vi "read groundwater header csv file.vi"(4 "Groundwater header file":path, 6 "header indicator reference 3":refnum<vi>, 7 "Groundwater Header":T1, 9 "Groundwater Cluster reference in":refnum<vi>, 10 "Read Groundwater Header File":bool, 11 "Sonde Serial Number String in":refnum<vi>) -> ()   [LabVIEW 2016]
uses:
  sdi_12/Groundwater header.ctl
  <vilib>/Utility/file.llb/Read Delimited Spreadsheet (string).vi
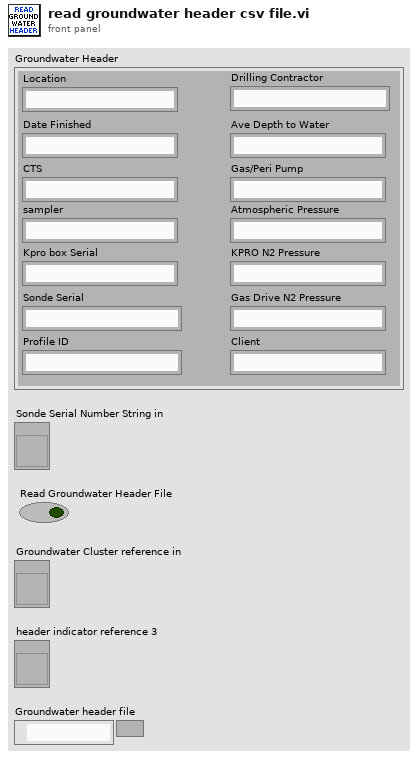
[diagram p1: front panel]
types:
  T1 = typedef "Groundwater header.ctl" = cluster{"Location":string, "Date Finished":string, "CTS":string, "sampler":string, "Kpro box Serial ":string, "Sonde Serial":string, "Drilling Contractor":string, "Ave Depth to Water":string, "Gas/Peri Pump":string, "Atmospheric Pressure":string, "KPRO N2 Pressure":string, "Gas Drive N2 Pressure":string, "Profile ID":string, "Client":string}
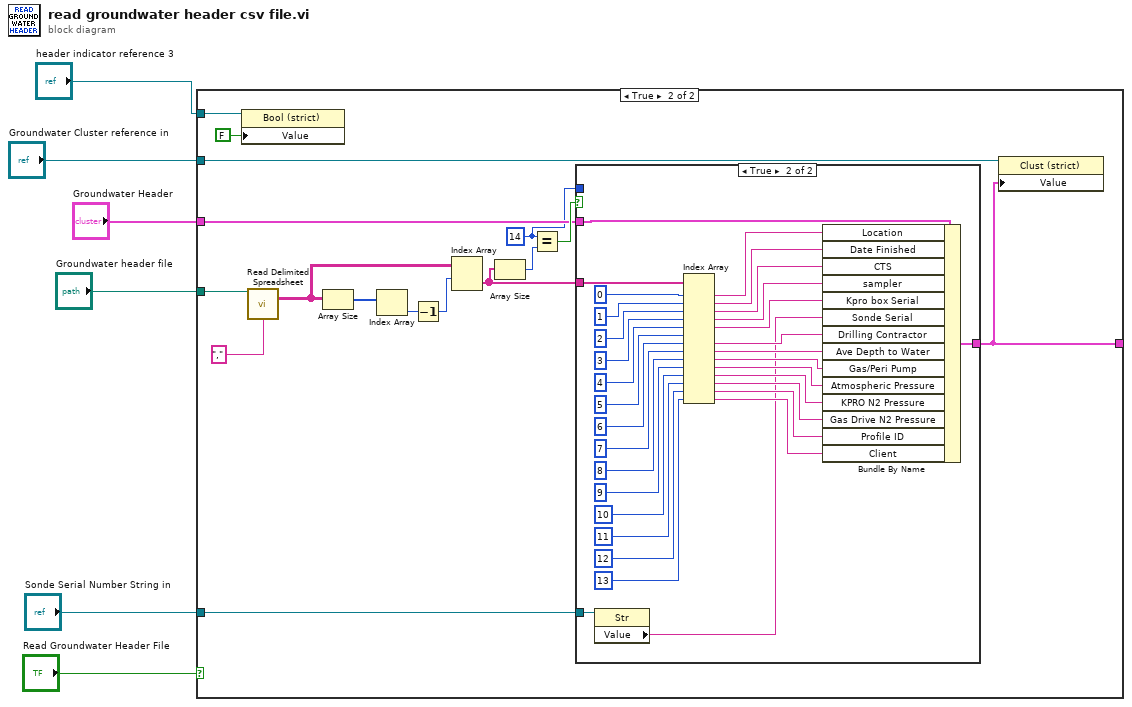
[diagram p0: block diagram]
diagram:
  n1 = case shown="True" "Read Groundwater Header File" {
    tunnel: "Groundwater Header" -> [w7 w19]
    tunnel: [w7 w18] -> _
    tunnel: "Groundwater header file" -> [_ w23]
    tunnel: "Sonde Serial Number String in" -> [_ w10]
    tunnel: "Groundwater Cluster reference in" -> [_ w9]
    tunnel: "header indicator reference 3" -> [_ w8]
    frame False {
    }
    frame True {
      w16 = 14 ("x")
      n2 = property class="Bool (strict)"(reference=w8, "Value"=FALSE ("Read Groundwater Header File")) -> ()  [unwired: 1 in, 2 out]
      n3 = call-poly <vilib>:"Read Delimited Spreadsheet.vi"("file path (dialog if empty)"=w23, "delimiter (\\t)"="," ("delimiter (\\t)")) -> ("all rows"=w13:string[][])  [unwired: 8 in, 5 out]
      n4 = Array Size(array=w13) -> (size(s)=w15:i32[])
      n5 = Index Array(array=w15) -> (element=w14:i32)  [unwired: 1 in]
      n6 = Decrement(x=w14) -> (x-1=w12:i32)
      n7 = Index Array(array=w13, index (row)=w12) -> (element=w11:string[])  [unwired: 1 in]
      n8 = Array Size(array=w11) -> (size(s)=w21:i32)
      n9 = Equal?(x=w16, y=w21) -> (x = y?=w20:bool)
      n10 = case shown="True" w20 {
        tunnel: w11 -> [_ w54]
        tunnel: [w24 w55] -> w18
        tunnel: w19 -> [w24 w56]
        tunnel: w16 -> [_ _]
        tunnel: w10 -> [_ w25]
        frame False {
        }
        frame True {
          n11 = property class="Str"(reference=w25) -> ("Value"=w26:string)  [unwired: 1 in, 2 out]
          n12 = Index Array(array=w54, index #1=0 ("index"), index #2=1 ("index"), index #3=2 ("index"), index #4=3 ("index"), index #5=4 ("index"), index #6=5 ("index"), index #7=6 ("index"), index #8=7 ("index"), index #9=8 ("index"), index #10=9 ("index"), index #11=10 ("index"), index #12=11 ("index"), index #13=12 ("index"), index #14=13 ("index")) -> (element #1=w53:string, element #2=w50:string, element #3=w48:string, element #4=w44:string, element #5=w43:string, element #7=w42:string, element #8=w41:string, element #9=w40:string, element #10=w39:string, element #11=w38:string, element #12=w37:string, element #13=w36:string, element #14=w35:string)  [unwired: 1 out]
          n13 = Bundle By Name(cluster=w56, "Location"=w53, "Date Finished"=w50, "CTS"=w48, "sampler"=w44, "Kpro box Serial"=w43, "Sonde Serial"=w26, "Drilling Contractor"=w42, "Ave Depth to Water"=w41, "Gas/Peri Pump"=w40, "Atmospheric Pressure"=w39, "KPRO N2 Pressure"=w38, "Gas Drive N2 Pressure"=w37, "Profile ID"=w36, "Client"=w35) -> (w55:T1)
        }
      }
      n14 = property class="Clust (strict)"(reference=w9, "Value"=w18) -> ()  [unwired: 1 in, 2 out]
    }
  }
